vi "CoerceTest.vi"() -> ()   [LabVIEW 2015]
panel:
  in  "stop":bool
  in  "Slide":dbl(slide) scale=-5.0..5.0
  out "coerced(x)":dbl
  in  "lower limit":dbl
  in  "upper limit":dbl
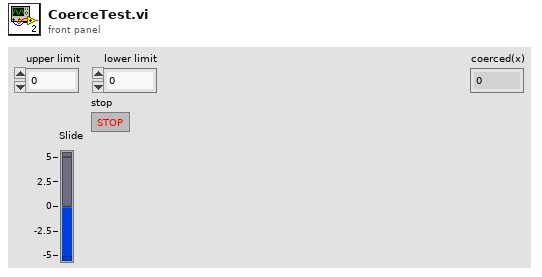
[diagram p1: front panel]
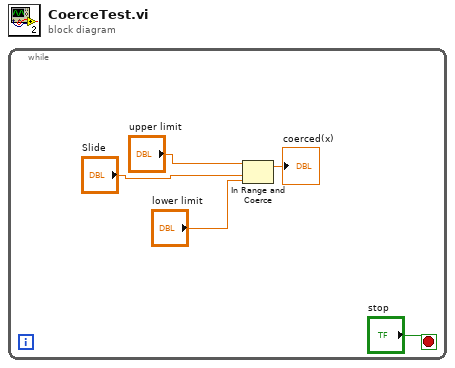
[diagram p0: block diagram]
diagram:
  n1 = while {
    stop <- "stop" stop-if-true
    n2 = In Range and Coerce(upper limit="upper limit", x="Slide", lower limit="lower limit") -> (coerced(x)=→"coerced(x)":dbl)  [unwired: 1 out]
  }
